vi "Generate Trace.vi"(11 "String":string) -> ()   [LabVIEW 2020, in "Actor Framework.lvlib"]
uses:
  Actor Framework.lvlib
  Inspection API/AF Trace Format/AF Trace Format.lvclass
  <resource>/dialog/lvconfig.llb/LV Config Read String.vi
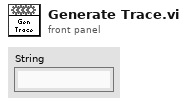
[diagram p1: front panel]
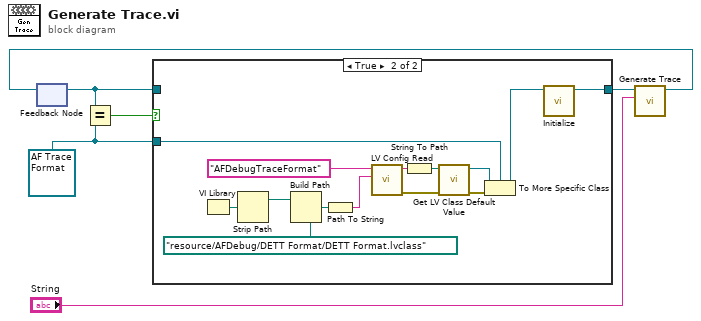
[diagram p0: block diagram]
diagram:
  w2 = refnum<class "AF Trace Format.lvclass"> refnum ("Actor Framework:AF Trace Format.lvclass")
  n1 = feedback #1() -> (w5:refnum<class "AF Trace Format.lvclass">)  [unwired: 1 in]
  n2 = Equal?(x=w5, y=w2) -> (x = y?=w4:bool)
  n3 = case shown="True" w4 {
    tunnel: w5 -> [w7 _]
    tunnel: [w7 w8] -> w3
    tunnel: w2 -> [_ w10]
    frame False {
    }
    frame True {
      n4 = VI Library() -> (path=w20:path)
      n5 = Strip Path(path=w20) -> (stripped path=w19:path)  [unwired: 1 out]
      n6 = Build Path(base path=w19, name or relative path=path "resource/AFDebug/DETT Format/DETT Format.lvclass") -> (appended path=w17:path)
      n7 = Path To String(path=w17) -> (string=w16:string)
      n8 = call-poly <resource>:"LV Config Read.vi"("default value"=w16, "key"="AFDebugTraceFormat") -> ("error out"=w15:errorcluster, "value"=w13:string)  [unwired: 3 in, 1 out]
      n9 = String To Path(string=w13) -> (path=w14:path)
      n10 = call <vilib>:"Get LV Class Default Value.vi"("error in (no error)"=w15, "class path"=w14) -> ("error out"=w12:errorcluster, "object"=w11:refnum<class>)  [unwired: 8 in]
      n11 = To More Specific Class(target class=w10, reference=w11, error in=w12) -> (specific class reference=w9:refnum<class "AF Trace Format.lvclass">)  [unwired: 1 out]
      n12 = call-dynamic "Initialize.vi"("AF Trace Format in"=w9) -> ("AF Trace Format out"=w8:refnum<class "AF Trace Format.lvclass">)  [unwired: 9 in, 1 out]
    }
  }
  n13 = call-dynamic "Generate Trace.vi"("Trace String"="String", "AF Trace Format in"=w3) -> ("AF Trace Format out"=w1:refnum<class "AF Trace Format.lvclass">)  [unwired: 9 in]
  n14 = feedback-in #1(w1) -> ()
